vi "Initialize IO.vi"(8 "error in":errorcluster, 11 "PLC in":refnum<class "PLC.lvclass">) -> (0 "error out":errorcluster, 3 "PLC out":refnum<class "PLC.lvclass">)   [LabVIEW 2018, in "PLC.lvlib" / "PLC.lvclass"]
uses:
  PLC.lvclass
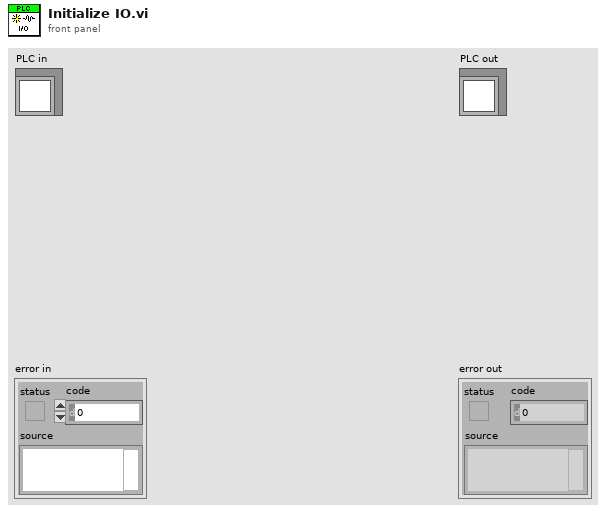
[diagram p1: front panel]
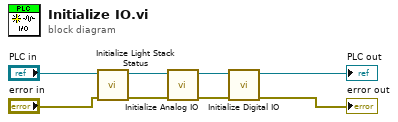
[diagram p0: block diagram]
diagram:
  n1 = call "Initialize Light Stack Status.vi"("error in"="error in", "PLC in"="PLC in") -> ("error out"=w3:errorcluster, "PLC out"=w4:refnum<class "PLC.lvclass">)  [unwired: 8 in]
  n2 = call "Initialize Analog IO.vi"("error in"=w3, "PLC in"=w4) -> ("error out"=w7:errorcluster, "PLC out"=w8:refnum<class "PLC.lvclass">)  [unwired: 8 in]
  n3 = call "Initialize Digital IO.vi"("error in"=w7, "PLC in"=w8) -> ("error out"=→"error out":errorcluster, "PLC out"=→"PLC out":refnum<class "PLC.lvclass">)  [unwired: 8 in]
